vi "read.vi"(8 "error in (no error)":errorcluster, 11 "Lakeshore 218 in":refnum<class "Lakeshore 218.lvclass">) -> (0 "error out":errorcluster, 2 "Data":dbl[](array[numeric]), 3 "Lakeshore 218 out":refnum<class "Lakeshore 218.lvclass">)   [LabVIEW 2022 SP3, in "Lakeshore 218.lvclass"]
uses:
  Lakeshore 218.lvclass
  Lakeshore 218.lvclass/Lakeshore 218.ctl
  <instrlib>/Lake Shore Cryotronics 218/Lake Shore Cryotronics 218.lvlib
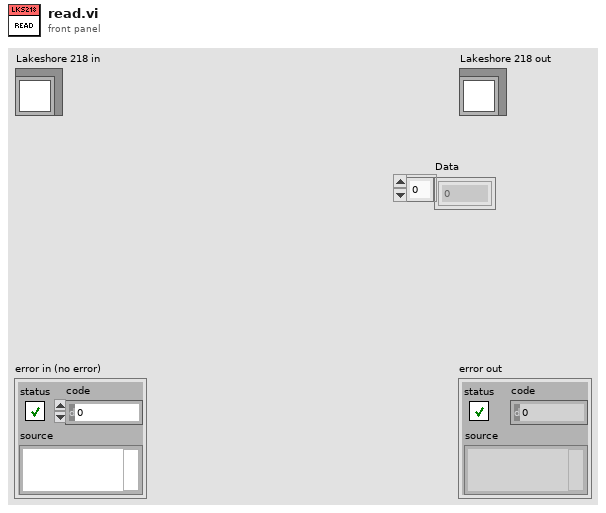
[diagram p1: front panel]
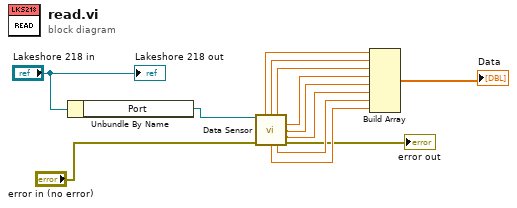
[diagram p0: block diagram]
diagram:
  n1 = Unbundle By Name("Lakeshore 218 in") -> ("Port"=w13:refnum<visa-resource-name>)
  n2 = call <instrlib>:"Data Sensor.vi"("VISA resource name"=w13, "error in (no error)"="error in (no error)") -> ("Input 1"=w11:dbl, "Input 2"=w10:dbl, "Input 3"=w9:dbl, "Input 4"=w8:dbl, "Input 5"=w7:dbl, "Input 6"=w6:dbl, "Input 8"=w4:dbl, "Input 7"=w5:dbl, "error out"=→"error out":errorcluster)  [unwired: 4 in, 1 out]
  n3 = Build Array(w11, w10, w9, w8, w7, w6, w5, w4) -> (→"Data":dbl[])
  "Lakeshore 218 out" <- "Lakeshore 218 in"
